vi "FPGA-HS-Parallel-Port-Receiver-Endless.vi"() -> ()   [LabVIEW 2016]
uses:
  <vilib>/Platform/TimedLoop/XDataNode/timing_clust.ctl
  <vilib>/Platform/TimedLoop/XDataNode/nitl_modes.ctl
  <vilib>/Platform/TimedLoop/XDataNode/wakeup.ctl
  <vilib>/rvi/Emulation/niFpgaGetClockAttributes.vi
  <vilib>/rvi/Emulation/niFpgaSctlEmulationGetInTimedLoop.vi
  <vilib>/rvi/Emulation/niFpgaEmulationReportErrorSimple.vi
  <vilib>/rvi/Emulation/niFpgaCriticalErrorInLSC.vi
  <vilib>/rvi/eio/common/nirviEmuTemplateMethod_errors.vi
  <vilib>/rvi/Emulation/niFpgaProcessEmulError.vi
  <vilib>/Platform/TimedLoop/XDataNode/XDataNode.xnode
  <vilib>/eio/EIONode/EIONode.xnode
  <vilib>/Platform/TimedLoop/XDataNode/XDNodeRunTimeDep.lvlib
panel:
  out "NewVal":bool
  out "OldVal":bool
  in  "Play Button":bool
  out "CompareVal":u16
  out "OldVal":u16
  in  "StepSize":u16
  in  "CompArray":u16[](array[numeric])=[0, 1, 2, 3, 4, 5, 6, 7, 8, 9, 10, 11, 12, 13, 14, 15, 16, 17, 18, 19, 20, 21, 22, 23, 24, 25, 26, 27, 28, 29, 30, 31, 32, 33, 34, 35, 36, 37, 38, 39, 40, 41, 42, 43, 44, 45, 46, 47, 48, 49, 50, 51, 52, 53, 54, 55, 56, 57, 58, 59, 60, 61, 62, 63] format="%x"
  in  "StopOnError?":bool
  out "CurrentIndex":u16 format="%x"
  out "CurrentSample":u16 format="%x"
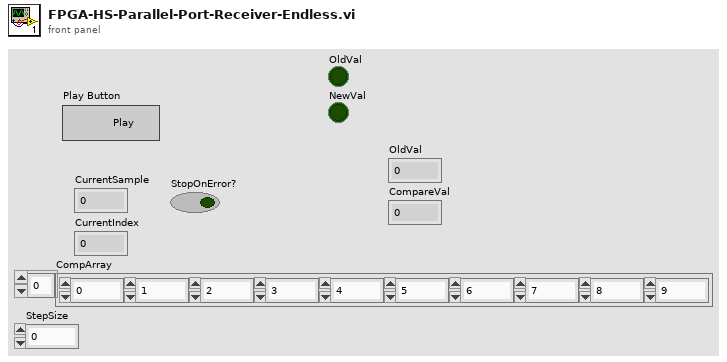
[diagram p1: front panel]
types:
  T1 = typedef "XDNodeRunTimeDep.lvlib/timing_clust.ctl" = cluster{"Expected End [f-1]":u64, "Actual End [f-1]":u64, "Finished Late? [f-1]":bool, "Expected End [i-1]":u64, "Actual End [i-1]":u64, "Finished Late? [i-1]":bool, "Expected Start [i]":u64, "Actual Start [i]":u64, "Expected Start [f]":u64, "Actual Start [f]":u64, "Source Name":string, "Structure Name":string, "Period":i64, "Deadline":i64, "Offset":i64, "Start":i64, "Priority":i32, "Timeout":i32, "Mode":T2, "Wakeup Reason":T3, "Error":errorcluster, "Source Type":string, "Secondary Source Type":string, "Global End Time":u64, "Global Start Time":u64, "Frame Duration":u64, "Iteration Duration":u64, "Assigned CPU":i32, "I/O Scan Engine Mode":u32}
  T2 = typedef "XDNodeRunTimeDep.lvlib/nitl_modes.ctl" = enum32{"No Change", "Process missed periods, maintain original phase", "Discard missed periods, maintain original phase", "Process missed periods, ignore original phase", "Discard missed periods, ignore original phase"}
  T3 = typedef "XDNodeRunTimeDep.lvlib/wakeup.ctl" = enum32{"Normal", "Aborted", "Asynchronous wakeup", "Timing source error", "Timed loop error", "Timeout"}
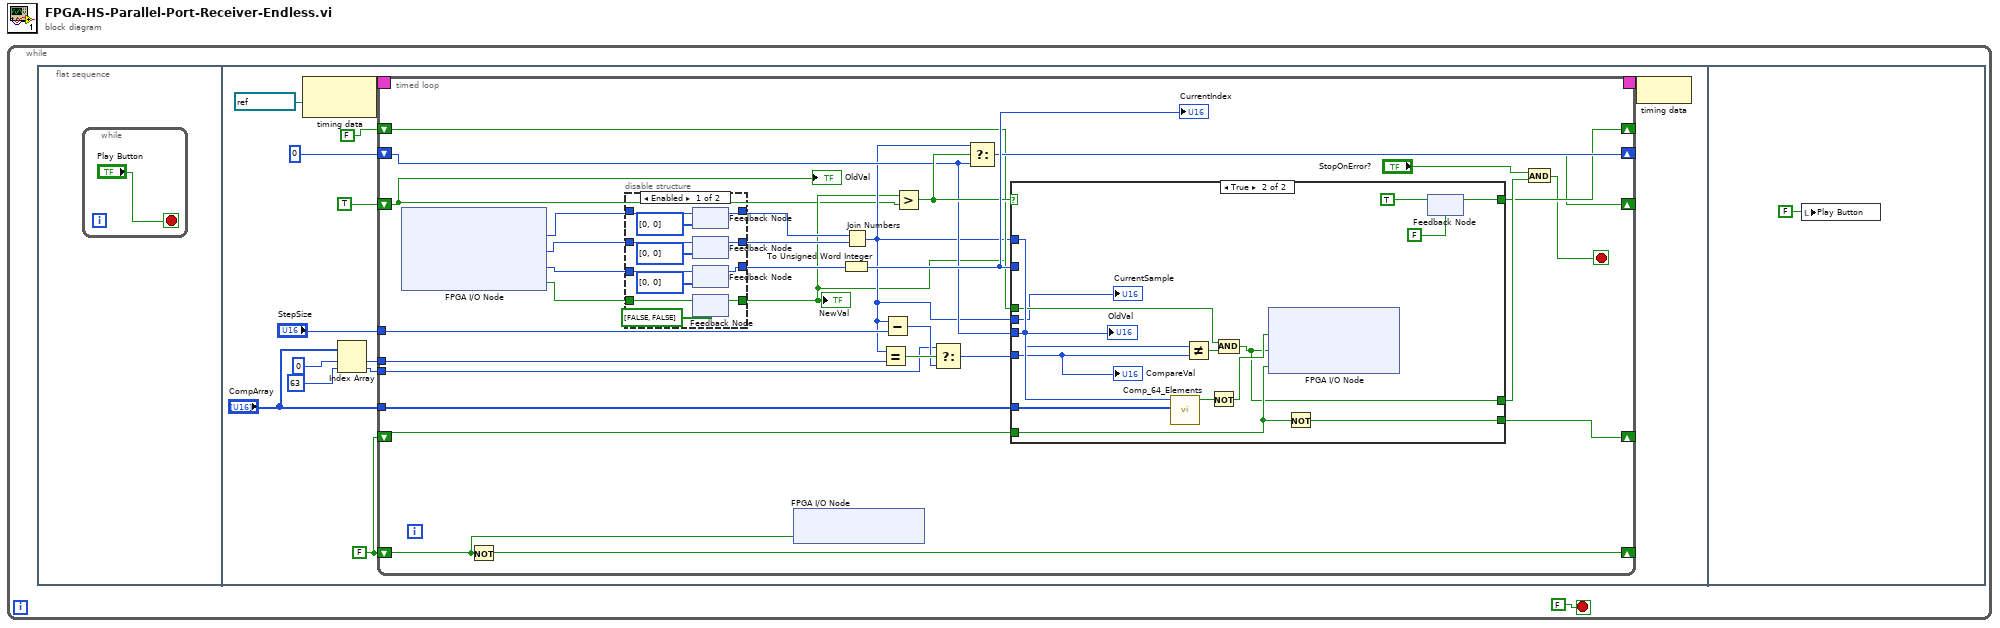
[diagram p0: block diagram]
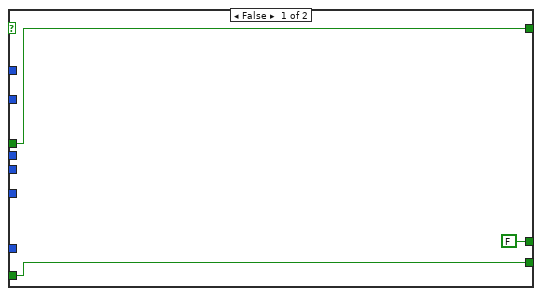
[diagram p3: hidden frame]
diagram:
  n1 = while {
    stop <- FALSE stop-if-true
    n2 = flat-sequence {
      frame #0 {
        n3 = while {
          stop <- "Play Button" stop-if-true
        }
      }
      frame #1 {
        w3 = FALSE ("ConnectorB/DIO8")
        n4 = node-c288(refnum<k21> "30MHz" ("Source Name")) -> (w15:T1)
        n5 = Index Array(array="CompArray", index #1=0 ("index"), index #2=63 ("index")) -> (element #1=w7:u16, element #2=w6:u16)
        n6 = timed-loop {
          timing: w15 -> [_]
          timing-out: [_] -> w14
          shift-right: [w17] -> _
          shift-left: TRUE ("ConnectorB/DIO8") -> [w16]
          shift-right: [w41] -> _
          shift-left: w3 -> [w37]
          tunnel: "CompArray" -> [w35]
          tunnel: "StepSize" -> [w32]
          shift-right: [w29] -> _
          shift-left: u16 0 -> [w27]
          tunnel: w7 -> [w31]
          tunnel: w6 -> [w30]
          shift-right: [w25] -> _
          shift-left: FALSE -> [w26]
          shift-right: [w23] -> _
          shift-left: w3 -> [w24]
          stop <- w21 stop-if-true
          n7 = xnode "FPGA I/O Node"() -> ("ConnectorA/DIO15:8"=w45:u8, "ConnectorA/DIO7:0"=w44:u8, "ConnectorB/DIO7:0"=w43:u8, "ConnectorB/DIO8"=w42:bool)  [unwired: 4 in, 4 out]
          n8 = Not(x=w37) -> (.not. x?=w41:bool)
          n9 = disable-structure shown="Enabled" {
            disable-tunnel: w45 -> [w57 w61]
            disable-tunnel: w44 -> [w56 w60]
            disable-tunnel: w43 -> [w55 w59]
            disable-tunnel: w42 -> [w54 w58]
            disable-tunnel: [w53 w61] -> w20
            disable-tunnel: [w52 w60] -> w19
            disable-tunnel: [w51 w59] -> w18
            disable-tunnel: [w50 w58] -> w17
            frame Enabled {
              n10 = feedback #1(u8[] [0, 0]) -> (w53:u8)
              n11 = feedback-in #1(w57) -> ()
              n12 = feedback #2(u8[] [0, 0]) -> (w52:u8)
              n13 = feedback-in #2(w56) -> ()
              n14 = feedback #3(u8[] [0, 0]) -> (w51:u8)
              n15 = feedback-in #3(w55) -> ()
              n16 = feedback #4(bool[] [FALSE, FALSE]) -> (w50:bool)
              n17 = feedback-in #4(w54) -> ()
            }
            frame Disabled {
            }
          }
          "NewVal" <- w17
          n18 = xnode "FPGA I/O Node"("ConnectorC/DIO7"=w37) -> ()  [unwired: 1 in, 1 out]
          n19 = To Unsigned Word Integer(number=w18) -> (unsigned 16bit integer=w39:u16)
          "CurrentIndex" <- w39
          n20 = Join Numbers(hi=w20, lo=w19) -> ((hi.lo)=w22:u16)
          n21 = Equal?(x=w22, y=w31) -> (x = y?=w34:bool)
          n22 = Subtract(x=w22, y=w32) -> (x-y=w33:u16)
          n23 = Greater?(x=w17, y=w16) -> (0:w28:bool)
          n24 = Select(t=w30, s=w34, f=w33) -> (s? t:f=w36:u16)
          n25 = Select(t=w22, s=w28, f=w27) -> (s? t:f=w29:u16)
          n26 = case shown="True" w28 {
            tunnel: [FALSE w69] -> w38
            tunnel: w22 -> [_ w76]
            tunnel: w39 -> [_ _]
            tunnel: w35 -> [_ w77]
            tunnel: w36 -> [_ w74]
            tunnel: w27 -> [_ w75]
            tunnel: w26 -> [w64 w72]
            tunnel: [w64 w67] -> w25
            tunnel: w24 -> [w63 w70]
            tunnel: [w63 w71] -> w23
            tunnel: w22 -> [_ w65]
            frame False {
            }
            frame True {
              n27 = call "Comp_64_Elements.vi"("Array"=w77, "CompVal"=w76) -> ("Boolean"=w79:bool)  [unwired: 9 in]
              n28 = Not Equal?(x=w75, y=w74) -> (x != y?=w73:bool)
              n29 = Not(x=w79) -> (.not. x?=w78:bool)
              n30 = And(x=w72, y=w73) -> (x .and. y?=w69:bool)
              n31 = xnode "FPGA I/O Node"("ConnectorC/DIO0"=w78, "ConnectorC/DIO1"=w69, "ConnectorC/DIO2"=w70) -> ()  [unwired: 3 in, 3 out]
              n32 = Not(x=w70) -> (.not. x?=w71:bool)
              n33 = feedback-in #5(TRUE) -> ()
              n34 = feedback #5(FALSE) -> (w67:bool)
              "CurrentSample" <- w65
              "OldVal" <- w75
              "CompareVal" <- w74
            }
          }
          n35 = And(x="StopOnError?", y=w38) -> (x .and. y?=w21:bool)
          "OldVal" <- w16
        }
        n36 = node-c288(w14) -> ()
      }
      frame #2 {
        n37 = local write "Play Button"(FALSE ("Play Button")) -> ()
      }
    }
  }
